vi "Read Object Name.vi"(8 "error in (no error)":errorcluster, 11 "Base in":refnum<class "CS++Base.lvclass">) -> (0 "error out":errorcluster, 2 "Object Name":string, 3 "Base out":refnum<class "CS++Base.lvclass">)   [LabVIEW 2012, in "CS++BaseClasses.lvlib" / "CS++Base.lvclass"]
doc: "Read name of object."
uses:
  CS++Base.lvclass
  CS++Base.lvclass/CS++Base.ctl
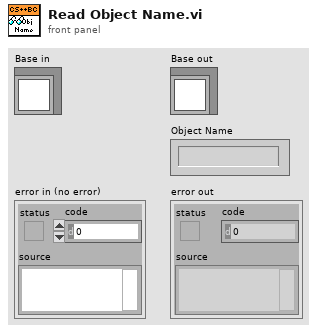
[diagram p1: front panel]
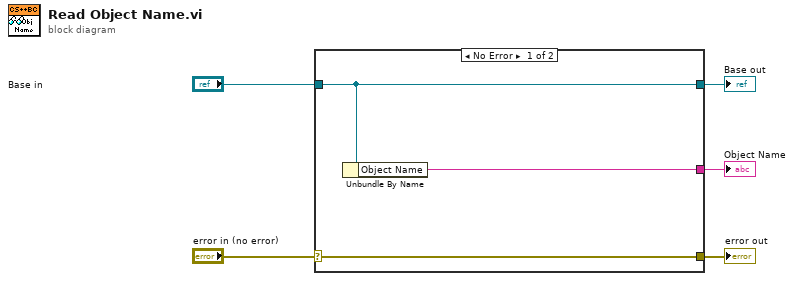
[diagram p0: block diagram]
diagram:
  n1 = case shown="No Error" "error in (no error)" {
    selector: "error in (no error)" -> [w8 w9]
    tunnel: [w8 w9] -> w4
    tunnel: [w7 w10] -> w2
    tunnel: "Base in" -> [w7 w10]
    tunnel: [w6 _] -> w1
    frame No Error {
      n2 = Unbundle By Name(w7) -> ("Object Name"=w6:string)
    }
    frame Error {
    }
  }
  "error out" <- w4
  "Base out" <- w2
  "Object Name" <- w1
